vi "Begin.vi"() -> ()   [LabVIEW 2016]
doc: "Called before other user functions, this VI is expected to open initial I/O refnums, load in file data, and do all program initialization. Notice that the <B>error out</B> terminal is simply used for data flow. Wiring it to other structures or subVIs ensures that this VI runs first."
uses:
  Refname/Swerve Motors.ctl
  Refname/Drive Motors.ctl
  Refname/Other Motors.ctl
  Refname/Controllers.ctl
  <vilib>/Rock Robotics/WPI/Joystick/WPI_JoystickDeviceEnum.ctl
  Refname/Huskie Board.ctl
  <vilib>/Rock Robotics/WPI/ThirdParty/Sensors/Huskie Board/LED Channels.ctl
  Refname/Sensors.ctl
  <vilib>/Rock Robotics/SystemInterfaces/spilib/spi_bus.ctl
  <vilib>/Rock Robotics/WPI/ThirdParty/CanMotor/TalonSRX/WPI_CANTalonSRX_APIControlMode.ctl
  <vilib>/Rock Robotics/WPI/SafetyOutput/WPI_SafetyOutputConfigMenu.ctl
  <vilib>/Rock Robotics/WPI/ThirdParty/CanMotor/TalonSRX/WPI_CANTalonSRX_APIFeedbackSelect.ctl
  Refname/Refname to String (Drive).vi
  Refname/Refname to String (Swerve).vi
  Refname/Refname to String (Other Motors).vi
  Refname/Refname to String (Controllers).vi
  Refname/Refname to String (Huskie Board).vi
  Refname/Refname to String (Sensors).vi
  <vilib>/Rock Robotics/WPI/ThirdParty/Sensors/ADIS16448 IMU/ADIS16448_IMU.lvlib
panel:
  out "error out":errorcluster
  in  "Values to Log":string="TimeStamp, Teleop Called Times, X, Y, Z, a, b, c, d, setpoint 1, setpoint 2, setpoint 3, setpoint 4, wheel power 1, wheel power 2, wheel power 3, wheel power 4"
  in  "error in":errorcluster
  in  "PID gains":T1={"proportional gain (Kc)"=5.0, "integral time (Ti, min)"=0.032, "derivative time (Td, min)"=0.0} {"derivative time (Td, min)" format="%.3f"; "integral time (Ti, min)" format="%.8f"; "proportional gain (Kc)" format="%.8f"}
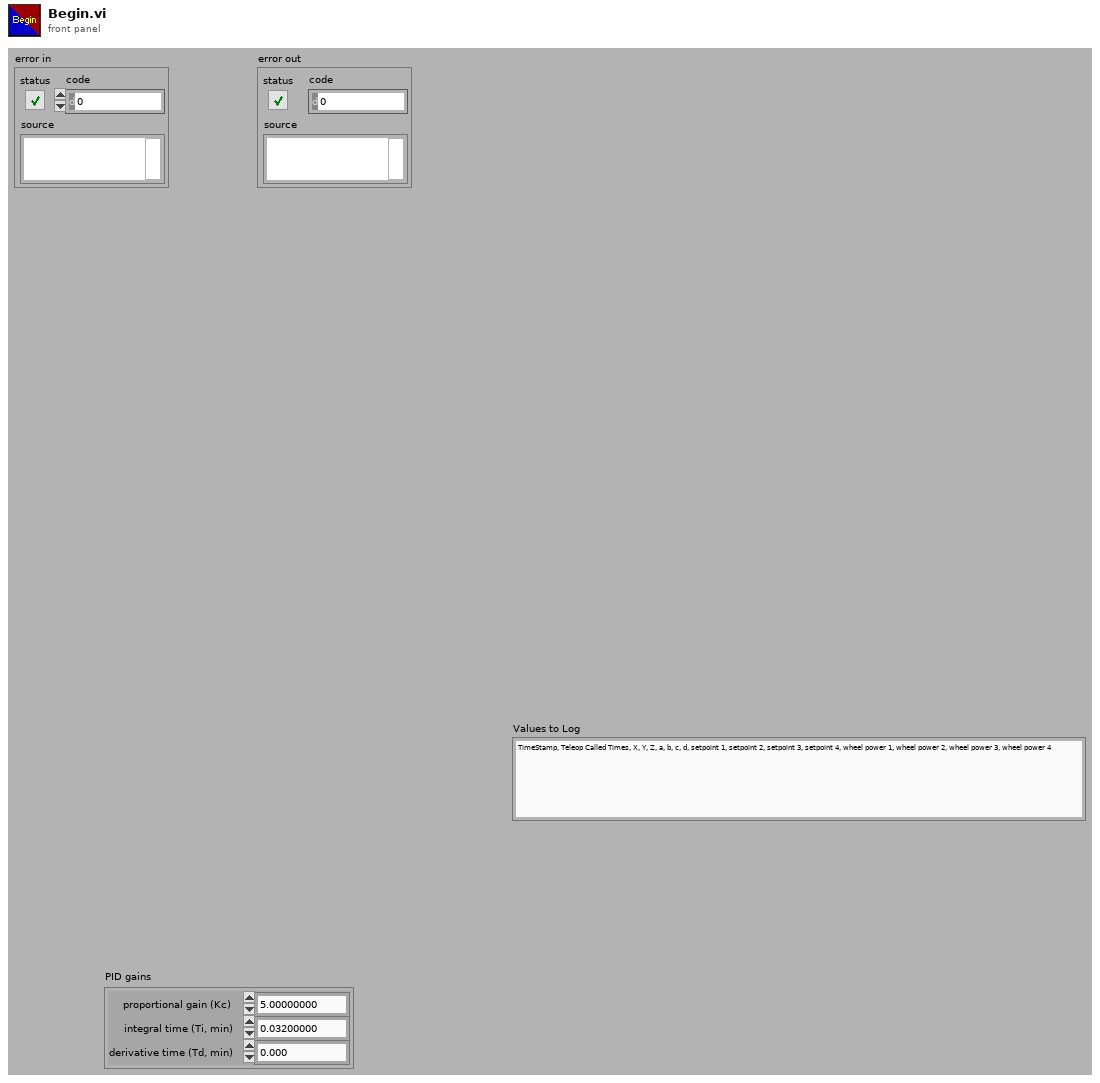
[diagram p1: front panel]
types:
  T1 = cluster{"proportional gain (Kc)":dbl, "integral time (Ti, min)":dbl, "derivative time (Td, min)":dbl}
  T2 = typedef "spi_bus.ctl" = enum16{"SPI On-Board, CS0", "SPI On-Board, CS1", "SPI On-Board, CS2", "SPI On-Board, CS3", "SPI MXP", "Invalid"}
  T3 = typedef "Sensors.ctl" = enum16{"Gyro", "Measure the thing", "Button Pressed", "Other sensor", "Generic Sensor"}
  T4 = typedef "Huskie Board.ctl" = enum16{"Huskie Board", "Log Queue", ""}
  T5 = typedef "LED Channels.ctl" = enum8{"SD card D1", "SD card D0", "SD card CLK", "SD card CMD", "SD card D2", "SD card D3", "roboRIO MOSI", "roboRIO MISO", "roboRIO CLK", "roboRIO CS", "roboRIO UART RX", "roboRIO UART TX", "roboRIO SCL", "robotRIO SDA", "HB GPIO 0", "HB GPIO 1", "HB GPIO 2", "HB GPIO 3", "HB LCD", "ADC CS2", "ADC CS1", "ADC DO", "ADC CLK", "ADC DI", "LED 1", "LED 2", "LED 3", "LED 4", "EEPROM SCL", "EEPROM SDA", "USB UART TX", "USB UART RX"}
  T6 = typedef "WPI_JoystickDeviceEnum.ctl" = enum16{"USB 0", "USB 1", "USB 2", "USB 3", "USB 4", "USB 5"}
  T7 = typedef "Controllers.ctl" = enum16{"Controller 0", "Controller 1", "Controller 2"}
  T8 = typedef "Other Motors.ctl" = enum16{"Climber", "Other motor", "Random Motor", "Spinny thingamajig", "Moves some blobs"}
  T9 = typedef "Drive Motors.ctl" = enum16{"Drive 1", "Drive 2", "Drive 3", "Drive 4"}
  T10 = typedef "Swerve Motors.ctl" = enum16{"Swerve 1", "Swerve 2", "Swerve 3", "Swerve 4"}
  T11 = typedef "WPI_CANTalonSRX_APIFeedbackSelect.ctl" = enum16{"Digital Quadrature Encoder", "Analog Potentiometer", "Analog Encoder", "Count on Quad-A (Rising-Edge)", "Count on Quad-A (Falling-Edge)", "CTR Magnetic Enc (Absolute)", "CTR Magnetic Enc (Relative)", "Pulse Width"}
  T12 = typedef "WPI_SafetyOutputConfigMenu.ctl" = enum16{"Enable", "Disable"}
  T13 = typedef "WPI_CANTalonSRX_APIControlMode.ctl" = enum8{"Percent VBus", "Speed", "Position", "Slave", "Unchanged / Invalid", "Voltage Compensation", "Current", "Motion Profile", "Motion Magic"}
  T14 = typedef "WPI_MotorControlDeviceRef.ctl" = cluster{"DeviceStatus":errorcluster, "Type":T15, "PWM":cluster{"PWM Channel":T16, "DeadBand":T17}, "CAN":cluster{"Device Number":u8, "SetOutput VI Ref":variant, "GetOutput VI Ref":variant, "Enable VI Ref":variant, "Disable VI Ref":variant, "Data":variant}, "Invert":bool}
  T15 = typedef "WPI_MotorControlType.ctl" = enum16{"PWM", "CAN"}
  T16 = typedef "FPGA_DIOPWMChannel.ctl" = enum8{"PWM 0", "PWM 1", "PWM 2", "PWM 3", "PWM 4", "PWM 5", "PWM 6", "PWM 7", "PWM 8", "PWM 9", "PWM MXP 0", "PWM MXP 1", "PWM MXP 2", "PWM MXP 3", "PWM MXP 4", "PWM MXP 5", "PWM MXP 6", "PWM MXP 7", "PWM MXP 8", "PWM MXP 9", "Invalid"}
  T17 = typedef "WPI_PWMDeadband.ctl" = cluster{"Name":string, "maxPositivePwm":i32, "minPositivePwm":i32, "centerPwm":i32, "maxNegativePwm":i32, "minNegativePwm":i32, "angularRange":u16}
  T18 = typedef "WPI_JoystickDevRef.ctl" = cluster{"Device":T6}
  T19 = typedef "ADIS16448_IMU.lvlib/ADI_IMU_ADIS16448_InterruptDevRef.ctl" = cluster{"ADI IMU DevRef":T20, "InterruptRef":T21}
  T20 = typedef "ADIS16448_IMU.lvlib/ADI_IMU_ADIS16448_IMUDevRef.ctl" = cluster{"DevStatus":errorcluster, "Handle":i32, "SPI Bus":T2, "Device Found":bool, "Device Ready":bool, "Yaw Axis":enum16{"X", "Y", "Z"}, "AHRS Algorithm":enum16{"Complementary", "Madgwick"}, "Serial":u16, "Lot ID 2":u16, "Lot ID 1":u16, "Product ID":u16}
  T21 = typedef "WPI_InterruptRef.ctl" = cluster{"DevStatus":errorcluster, "InterruptIndex":T22}
  T22 = typedef "FPGA_InterruptIndex.ctl" = enum8{"0", "1", "2", "3", "4", "5", "6", "7", "Invalid"}
  T23 = typedef "WPI_SerialPortRef.ctl" = cluster{"DevStatus":errorcluster, "Serial Port Name":refnum<visa-resource-name>}
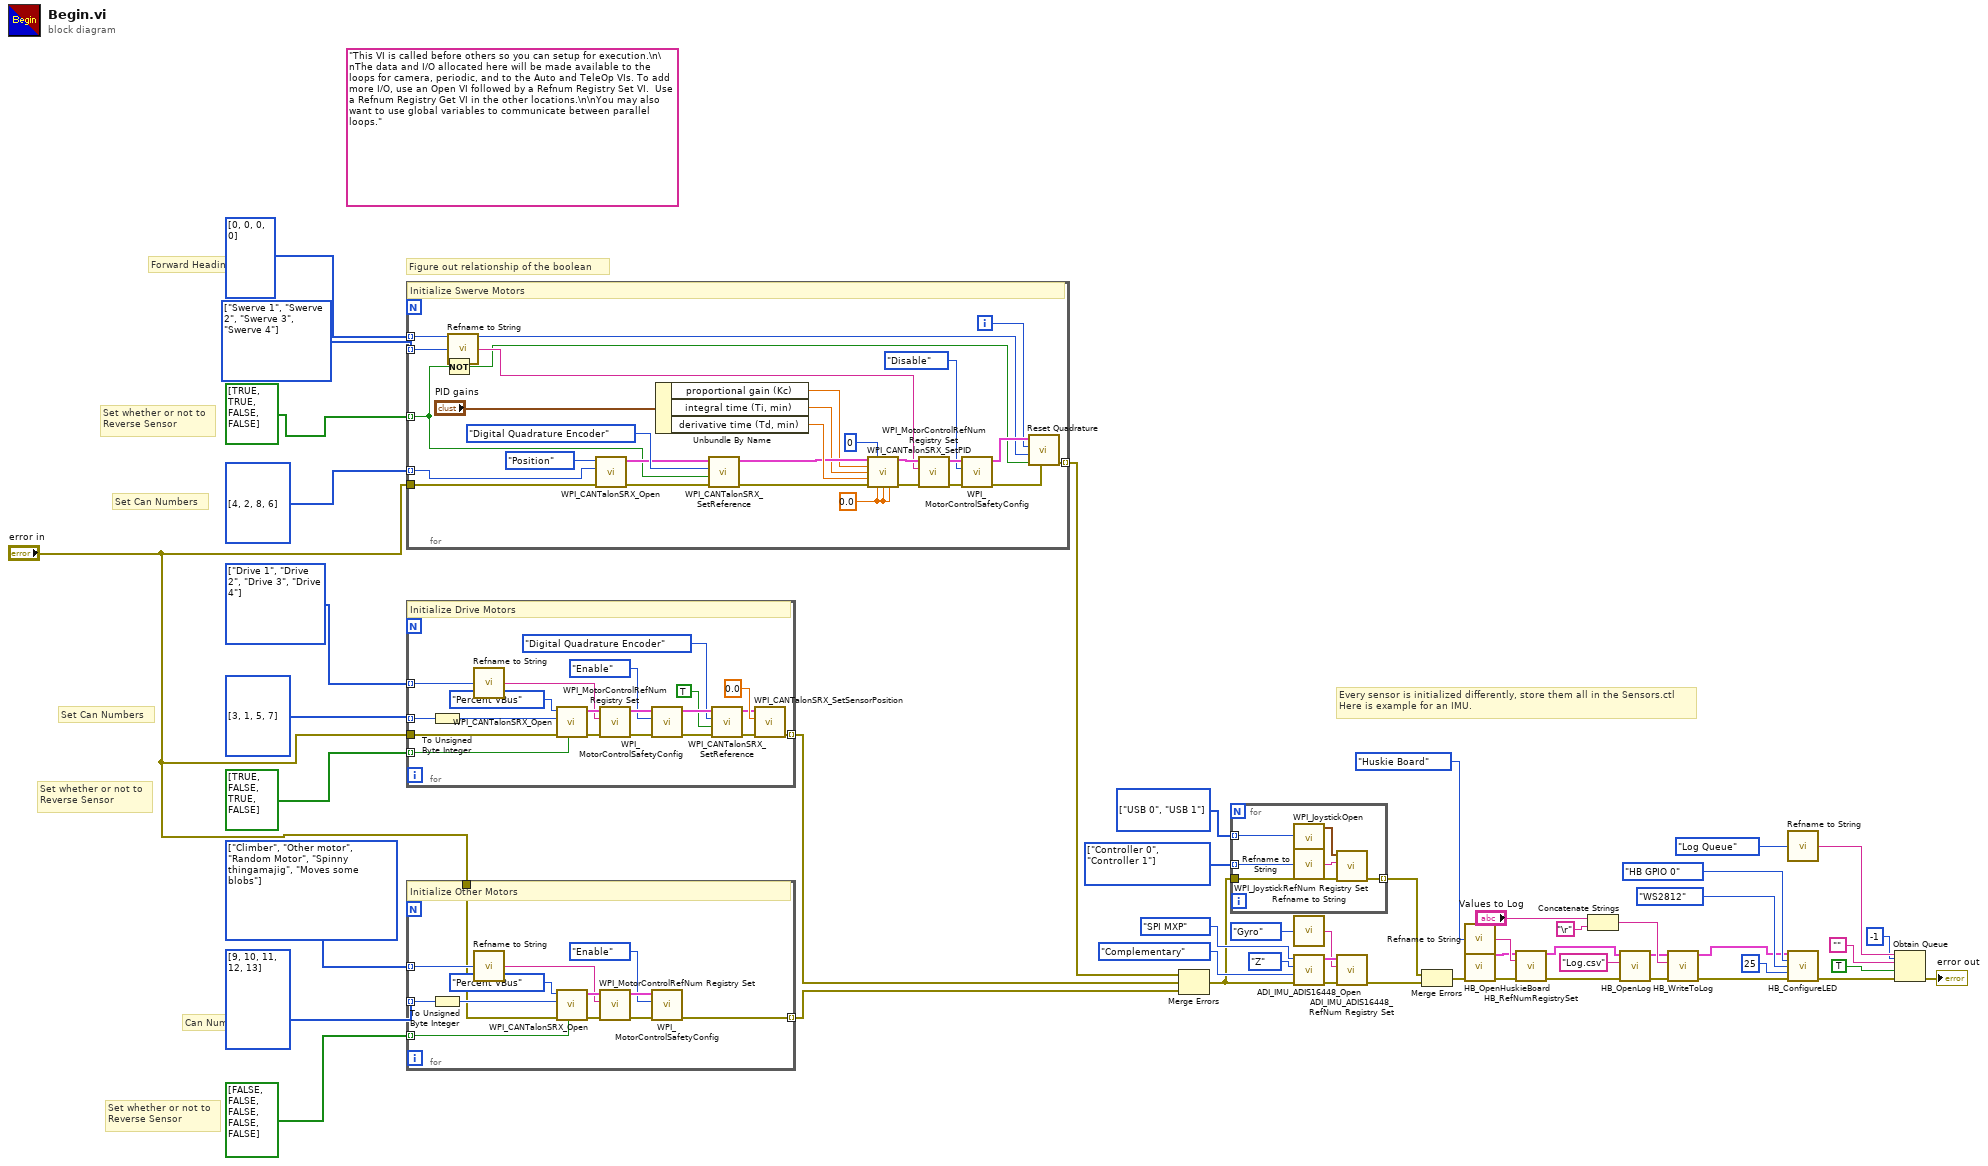
[diagram p0: block diagram]
diagram:
  w36 = T6[] [enum."USB 0", enum."USB 1"] items=["USB 0", "USB 1", "USB 2", "USB 3", "USB 4", "USB 5"]
  w37 = T7[] [enum."Controller 0", enum."Controller 1"] items=["Controller 0", "Controller 1", "Controller 2"]
  w44 = T8[] [enum."Climber", enum."Other motor", enum."Random Motor", enum."Spinny thingamajig", enum."Moves some blobs"] items=["Climber", "Other motor", "Random Motor", "Spinny thingamajig", "Moves some blobs"]
  w48 = T9[] [enum."Drive 1", enum."Drive 2", enum."Drive 3", enum."Drive 4"] items=["Drive 1", "Drive 2", "Drive 3", "Drive 4"]
  w49 = T10[] [enum."Swerve 1", enum."Swerve 2", enum."Swerve 3", enum."Swerve 4"] items=["Swerve 1", "Swerve 2", "Swerve 3", "Swerve 4"]
  (unwired) "This VI is called before others so you can setup for execution.\n\nThe data and I/O allocated here will be made available to the loops for camera, periodic, and to the Auto and TeleOp VIs. To add more I/O, use an Open VI followed by a Refnum Registry Set VI.  Use a Refnum Registry Get VI in the other locations.\n\nYou may also want to use global variables to communicate between parallel loops."
  # "Set whether or not to\nReverse Sensor"
  # "Set whether or not to\nReverse Sensor"
  # "Can Num"
  # "Forward Headings"
  # "Every sensor is initialized differently, store them all in the Sensors.ctl\nHere is example for an IMU."
  # "Figure out relationship of the boolean"
  # "Set Can Numbers"
  # "Set whether or not to\nReverse Sensor"
  # "Set Can Numbers"
  n1 = for {
    tunnel: i32[] [4, 2, 8, 6] -> [w62] mode=indexing
    tunnel: bool[] [TRUE, TRUE, FALSE, FALSE] -> [w55] mode=indexing
    tunnel: w49 -> [w61] mode=indexing
    tunnel: i32[] [0, 0, 0, 0] -> [w57] mode=indexing
    tunnel: "error in" -> [w53]
    tunnel: [w52] -> w40 mode=indexing
    i -> [w58]
    w70 = 0.0 ("Output")
    # "Initialize Swerve Motors"
    n2 = Not(x=w55) -> (.not. x?=w56:bool)
    n3 = call-poly "Refname to String.vi"("Enum"=w61) -> ("String"=w60:string)
    n4 = call <vilib>:"WPI_CANTalonSRX_Open.vi"("error in"=w53, "Device Number"=w62, "Control Mode"=WPI_CANTalonSRX_APIControlMode."Position") -> ("error out"=w73:errorcluster, "CAN Talon SRX Ref"=w74:T14)  [unwired: 7 in]
    n5 = Unbundle By Name("PID gains") -> ("proportional gain (Kc)"=w65:dbl, "integral time (Ti, min)"=w66:dbl, "derivative time (Td, min)"=w71:dbl)
    n6 = call <vilib>:"WPI_CANTalonSRX_SetReference.vi"("error in (no error)"=w73, "Reverse Feedback Sensor"=w55, "Feedback Reference"=WPI_CANTalonSRX_APIFeedbackSelect."Digital Quadrature Encoder", "CAN Talon SRX Ref"=w74) -> ("error out"=w68:errorcluster, "CAN Talon SRX Ref"=w69:T14)  [unwired: 6 in]
    n7 = call <vilib>:"WPI_CANTalonSRX_SetPID.vi"("CAN Talon SRX Ref"=w69, "Parameter Slot"=u8 0, "P"=w65, "I"=w66, "D"=w71, "error in (no error)"=w68, "F"=w70, "I Zone"=w70, "Ramp Rate"=w70) -> ("CAN Talon SRX Ref"=w63:T14, "error out"=w67:errorcluster)  [unwired: 5 in]
    n8 = call <vilib>:"WPI_MotorControlRefNum Registry Set.vi"("error in (no error)"=w67, "refnum name"=w60, "MotorControlDevRef"=w63) -> ("error out"=w78:errorcluster, "MotorControlDevRef"=w77:T14)  [unwired: 7 in]
    n9 = call <vilib>:"WPI_MotorControlSafetyConfig.vi"("error in (no error)"=w78, "mode"=WPI_SafetyOutputConfigMenu."Disable", "MotorControlDevRef"=w77) -> ("error out"=w54:errorcluster, "MotorControlDevRef"=w59:T14)  [unwired: 7 in]
    n10 = call "Reset Quadrature.vi"("error in"=w54, "Reverse?"=w56, "Forward Position"=w57, "Module Number"=w58, "CAN Talon SRX Ref"=w59) -> ("error out"=w52:errorcluster)  [unwired: 6 in]
  }
  n11 = for {
    tunnel: w48 -> [w84] mode=indexing
    tunnel: i32[] [3, 1, 5, 7] -> [w83] mode=indexing
    tunnel: bool[] [TRUE, FALSE, TRUE, FALSE] -> [w82] mode=indexing
    tunnel: "error in" -> [w81]
    tunnel: [w80] -> w39 mode=indexing
    # "Initialize Drive Motors"
    n12 = To Unsigned Byte Integer(number=w83) -> (unsigned 8bit integer=w92:u8)
    n13 = call-poly "Refname to String.vi"("Enum"=w84) -> ("resulting string"=w97:string)
    n14 = call <vilib>:"WPI_CANTalonSRX_Open.vi"("Invert"=w82, "error in"=w81, "Device Number"=w92, "Control Mode"=WPI_CANTalonSRX_APIControlMode."Percent VBus") -> ("error out"=w93:errorcluster, "CAN Talon SRX Ref"=w98:T14)  [unwired: 6 in]
    n15 = call <vilib>:"WPI_MotorControlRefNum Registry Set.vi"("error in (no error)"=w93, "refnum name"=w97, "MotorControlDevRef"=w98) -> ("error out"=w96:errorcluster, "MotorControlDevRef"=w95:T14)  [unwired: 7 in]
    n16 = call <vilib>:"WPI_MotorControlSafetyConfig.vi"("error in (no error)"=w96, "mode"=WPI_SafetyOutputConfigMenu."Enable", "MotorControlDevRef"=w95) -> ("error out"=w88:errorcluster, "MotorControlDevRef"=w87:T14)  [unwired: 7 in]
    n17 = call <vilib>:"WPI_CANTalonSRX_SetReference.vi"("error in (no error)"=w88, "Reverse Feedback Sensor"=TRUE, "Feedback Reference"=WPI_CANTalonSRX_APIFeedbackSelect."Digital Quadrature Encoder", "CAN Talon SRX Ref"=w87) -> ("error out"=w90:errorcluster, "CAN Talon SRX Ref"=w89:T14)  [unwired: 6 in]
    n18 = call <vilib>:"WPI_CANTalonSRX_SetSensorPosition.vi"("error in (no error)"=w90, "New Sensor Position"=0.0, "CAN Talon SRX Ref"=w89) -> ("error out"=w80:errorcluster)  [unwired: 7 in, 1 out]
  }
  n19 = for {
    tunnel: w44 -> [w104] mode=indexing
    tunnel: i32[] [9, 10, 11, 12, 13] -> [w103] mode=indexing
    tunnel: bool[] [FALSE, FALSE, FALSE, FALSE, FALSE] -> [w102] mode=indexing
    tunnel: "error in" -> [w101]
    tunnel: [w100] -> w38 mode=indexing
    # "Initialize Other Motors"
    n20 = To Unsigned Byte Integer(number=w103) -> (unsigned 8bit integer=w105:u8)
    n21 = call-poly "Refname to String.vi"("Enum"=w104) -> ("resulting string"=w110:string)
    n22 = call <vilib>:"WPI_CANTalonSRX_Open.vi"("Invert"=w102, "error in"=w101, "Device Number"=w105, "Control Mode"=WPI_CANTalonSRX_APIControlMode."Percent VBus") -> ("error out"=w106:errorcluster, "CAN Talon SRX Ref"=w111:T14)  [unwired: 6 in]
    n23 = call <vilib>:"WPI_MotorControlRefNum Registry Set.vi"("error in (no error)"=w106, "refnum name"=w110, "MotorControlDevRef"=w111) -> ("error out"=w109:errorcluster, "MotorControlDevRef"=w108:T14)  [unwired: 7 in]
    n24 = call <vilib>:"WPI_MotorControlSafetyConfig.vi"("error in (no error)"=w109, "mode"=WPI_SafetyOutputConfigMenu."Enable", "MotorControlDevRef"=w108) -> ("error out"=w100:errorcluster)  [unwired: 7 in, 1 out]
  }
  n25 = Merge Errors(w40, w39, w38) -> (w2:errorcluster)
  n26 = for {
    tunnel: w37 -> [w118] mode=indexing
    tunnel: w36 -> [w115] mode=indexing
    tunnel: w2 -> [w114]
    tunnel: [w113] -> w35 mode=indexing
    n27 = call <vilib>:"WPI_JoystickOpen.vi"("JoystickDevice"=w115) -> ("JoystickDevRef"=w117:T18)  [unwired: 10 in]
    n28 = call-poly "Refname to String.vi"("Enum"=w118) -> ("resulting string"=w116:string)
    n29 = call <vilib>:"WPI_JoystickRefNum Registry Set.vi"("error in (no error)"=w114, "refnum name"=w116, "JoystickDevRef"=w117) -> ("error out"=w113:errorcluster)  [unwired: 7 in, 1 out]
  }
  n30 = call-poly "Refname to String.vi"("Enum"=Sensors."Gyro") -> ("resulting string"=w5:string)
  n31 = call <vilib>:"ADI_IMU_ADIS16448_Open.vi"("error in"=w2, "AHRS Algorithm"=enum16{"Complementary", "Madgwick"}."Complementary", "Yaw Axis"=enum16{"X", "Y", "Z"}."Z", "SPI Chip Select"=spi_bus."SPI MXP") -> ("error out"=w9:errorcluster, "ADI IMU Interrupt DevRef"=w8:T19)  [unwired: 6 in]
  n32 = call <vilib>:"ADI_IMU_ADIS16448_RefNum Registry Set.vi"("error in (no error)"=w9, "refnum name"=w5, "ADI IMU Interrupt DevRef"=w8) -> ("error out"=w1:errorcluster)  [unwired: 7 in, 1 out]
  n33 = Merge Errors(w35, w1) -> (w18:errorcluster)
  n34 = call-poly "Refname to String.vi"("Enum"=Huskie_Board."Huskie Board") -> ("resulting string"=w20:string)
  n35 = call <vilib>:"HB_OpenHuskieBoard.vi"("error in (no error)"=w18) -> ("error out"=w33:errorcluster, "HBDeviceRef"=w19:T23)  [unwired: 9 in]
  n36 = call <vilib>:"HB_RefNumRegistrySet.vi"("HBDevRef"=w19, "refnum name"=w20, "error in (no error)"=w33) -> ("HBDevRef"=w21:T23, "error out"=w32:errorcluster)  [unwired: 11 in]
  n37 = Concatenate Strings("Values to Log", "\r") -> (w23:string)
  n38 = call <vilib>:"HB_OpenLog.vi"("error in (no error)"=w32, "File Name"="Log.csv", "HBDeviceRef"=w21) -> ("error out"=w31:errorcluster, "HBDeviceRef"=w22:T23)  [unwired: 7 in]
  n39 = call <vilib>:"HB_WriteToLog.vi"("error in (no error)"=w31, "Log string"=w23, "HBDevRef"=w22) -> ("error out"=w29:errorcluster, "HBDevRef"=w17:T23)  [unwired: 7 in]
  n40 = call-poly "Refname to String.vi"("Enum"=Huskie_Board."Log Queue") -> ("resulting string"=w15:string)
  n41 = call <vilib>:"HB_ConfigureLED.vi"("HBDevRef"=w17, "LED Strip Channel"=LED_Channels."HB GPIO 0", "LED Model"=enum8{"WS2812", "WS2812B"}."WS2812", "Number of LEDs"=u8 25, "error in (no error)"=w29) -> ("error out"=w11:errorcluster)  [unwired: 9 in, 1 out]
  n42 = Obtain Queue(max queue size (-1, unlimited)=-1, name (unnamed)=w15, element data type="", create if not found? (T)=TRUE, error in (no error)=w11) -> (error out=→"error out":errorcluster)  [unwired: 2 out]
